vi "Outtake for Time.vi"(6 "Synchronization":enum16{"Start", "Wait"}(ring), 7 "Description":string, 8 "Command Info In":T1, 10 "Duration (s)":dbl, 11 "Power":dbl) -> (0 "Command Info Out":T1)   [LabVIEW 2019]
doc: "This template has a parameter to control whether it waits for the command to complete or not. This is useful for operations that have a timed duration or a sensor-based duration. \n\nBe sure to right-click and select New from Template and save with a new command name."
uses:
  <vilib>/Rock Robotics/WPI/Framework/Command Status Info.ctl
  <vilib>/Rock Robotics/WPI/Framework/Completion Status.ctl
  <vilib>/Rock Robotics/WPI/Framework/Completion Notifier.ctl
  Implementation/Intake Setpoints.ctl
  Implementation/Intake Operations.ctl
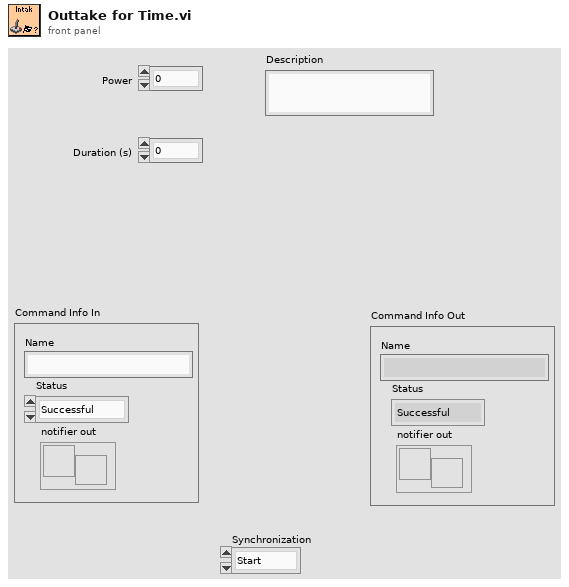
[diagram p1: front panel]
types:
  T1 = typedef "Command Status Info.ctl" = cluster{"Name":string, "Status":T2, "notifier out":T3}
  T2 = typedef "Completion Status.ctl" = enum16{"Successful", "Aborted", "Incomplete"}
  T3 = typedef "Completion Notifier.ctl" = refnum<notifier>
  T4 = typedef "Intake Setpoints.ctl" = cluster{"Operation":T5, "Power":dbl, "Duration":dbl}
  T5 = typedef "Intake Operations.ctl" = enum16{"Reserve", "Read Current", "Immediate", "Intake for Time", "Intake Immediate", "Outtake for Time", "Outtake Immediate"}
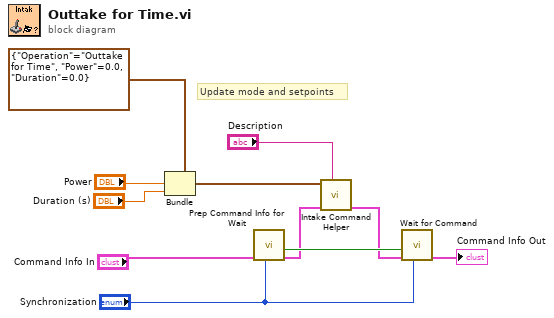
[diagram p0: block diagram]
diagram:
  # "Update mode and setpoints"
  n1 = Bundle(cluster=T4 {"Operation"=enum."Outtake for Time", "Power"=0.0, "Duration"=0.0} ("SubSystem Data"), "Power"="Power", "Duration"="Duration (s)") -> (w3:T4)  [unwired: 1 in]
  n2 = call <vilib>:"Prep Command Info for Wait.vi"("Synchronication"="Synchronization", "Command Info"="Command Info In") -> ("Command Info"=w7:T1, "Allocated"=w8:bool)  [unwired: 8 in]
  n3 = call "Intake Command Helper.vi"("Description"="Description", "Command Info In"=w7, "SubSystem Data"=w3) -> ("Command Info Out"=w4:T1)  [unwired: 6 in, 2 out]
  n4 = call <vilib>:"Wait for Command.vi"("Synchronication"="Synchronization", "Command Info in"=w4, "Allocated"=w8) -> ("Command Info out"=→"Command Info Out":T1)  [unwired: 8 in]
